vi "GetOutput.vi"(4 "error in":errorcluster, 5 "connection ID":refnum<k5>) -> (0 "Output":string, 1 "error out":errorcluster, 2 "connection ID out":refnum<k5>, 3 "Answer":bool)   [LabVIEW 2013]
panel:
  out "читаю hex":string
  out "читаю текст":string
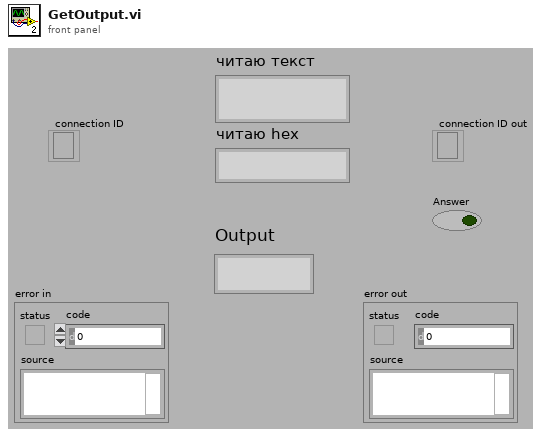
[diagram p1: front panel]
types:
  T1 = enum16{"Standard", "Buffered", "CRLF", "Immediate"}
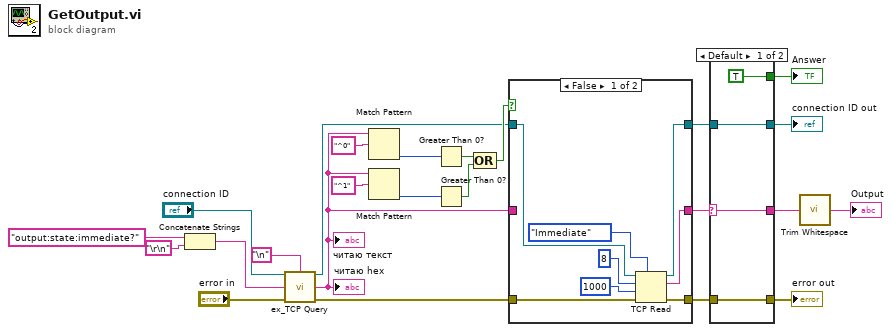
[diagram p0: block diagram]
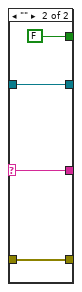
[diagram p3: hidden frame]
diagram:
  n1 = Concatenate Strings("output:state:immediate?" ("data in"), "\r\n") -> (w1:string)
  n2 = call "ex_TCP Query.vi"("TCP Network Connection in"="connection ID", "Termination character"="\n", "Query string"=w1, "error in (no error)"="error in") -> ("TCP Network Connection out"=w3:refnum<k5>, "Message data out"=w4:string, "error out"=w5:errorcluster)  [unwired: 8 in, 1 out]
  "читаю текст" <- w4
  "читаю hex" <- w4
  n3 = Match Pattern(string=w4, regular expression="^0") -> (offset past match=w18:i32)  [unwired: 1 in, 3 out]
  n4 = Match Pattern(string=w4, regular expression="^1") -> (offset past match=w20:i32)  [unwired: 1 in, 3 out]
  n5 = Greater Than 0?(x=w18) -> (x > 0?=w13:bool)
  n6 = Greater Than 0?(x=w20) -> (x > 0?=w12:bool)
  n7 = Compound Arithmetic op=OR(w13, w12) -> (w11:bool)
  n8 = case shown="False" w11 {
    tunnel: [w26 w35] -> w10
    tunnel: w3 -> [w25 w35]
    tunnel: w5 -> [w29 w34]
    tunnel: [w28 w34] -> w9
    tunnel: w4 -> [_ w33]
    tunnel: [w27 w33] -> w8
    frame False {
      n9 = TCP Read(connection ID=w25, bytes to read=8, error in (no error)=w29, 7:T1."Immediate" ("mode (standard)"), 9:1000 ("timeout ms (25000)")) -> (connection ID out=w26:refnum<k5>, data out=w27:string, error out=w28:errorcluster)
    }
    frame True {
    }
  }
  n10 = case shown="Default" w8 {
    selector: w8 -> [w39 w43]
    tunnel: [w39 w43] -> w22
    tunnel: [TRUE FALSE] -> w14
    tunnel: w9 -> [w37 w41]
    tunnel: [w37 w41] -> w16
    tunnel: w10 -> [w36 w40]
    tunnel: [w36 w40] -> w15
    frame Default {
    }
    frame "" {
    }
  }
  "Answer" <- w14
  "connection ID out" <- w15
  "error out" <- w16
  n11 = call <vilib>:"Trim Whitespace.vi"("string"=w22) -> ("trimmed string"=→"Output":string)  [unwired: 1 in]
